vi "Processing Loop.vi"   [LabVIEW 2014, in "navX Library v2.lvlib"]
uses:
  navX Library v2.lvlib
  TypeDefs/navX Device TypeDef.ctl
  TypeDefs/navX Protocol TypeDef.ctl
  TypeDefs/navX Notify Packet TypeDef.ctl
  TypeDefs/navX Action TypeDef.ctl
  <vilib>/Platform/TimedLoop/XDataNode/timing_clust.ctl
  <vilib>/Platform/TimedLoop/XDataNode/nitl_modes.ctl
  <vilib>/Platform/TimedLoop/XDataNode/wakeup.ctl
  <vilib>/platform/TimedLoop/XDataNode/XDataNode.xnode
  <vilib>/Platform/TimedLoop/XDataNode/XDNodeRunTimeDep.lvlib
types:
  T1 = typedef "navX Library v2.lvlib/navX Device TypeDef.ctl" = cluster{"Interface":cluster{"Protocol":T2, "Update Rate (4Hz-60Hz)":u8, "navX Open TypeDef":variant}, "Notifiy Packet":refnum<notifier>, "Loop VI Refnum":refnum<vi>}
  T2 = typedef "navX Library v2.lvlib/navX Protocol TypeDef.ctl" = enum16{"SERIAL", "I2C", "SPI"}
  T3 = typedef "navX Library v2.lvlib/navX Interface TypeDef.ctl" = cluster{"SerialPortRef":T4, "I2CDevRef":T5, "SPIDevRef":T8}
  T4 = typedef "WPI_SerialPortRef.ctl" = cluster{"DevStatus":errorcluster, "Serial Port Name":refnum<visa-resource-name>}
  T5 = typedef "WPI_I2CDevRef.ctl" = cluster{"DevStatus":errorcluster, "Controller":T6, "Device Address":u8, "Handle":i32, "I2C Bus":T7}
  T6 = typedef "FPGA_TypedefDigitalModule.ctl" = enum16{"Controller 1"}
  T7 = typedef "i2c_bus.ctl" = enum16{"I2C On-Board", "I2C MXP", "Invalid"}
  T8 = typedef "WPI_SPIDevRef.ctl" = cluster{"DevStatus":errorcluster, "Handle":i32, "Controller":T6, "SPI Bus":T9}
  T9 = typedef "spi_bus.ctl" = enum16{"SPI On-Board, CS0", "SPI On-Board, CS1", "SPI On-Board, CS2", "SPI On-Board, CS3", "SPI MXP", "Invalid"}
  T10 = typedef "XDNodeRunTimeDep.lvlib/timing_clust.ctl" = cluster{"Expected End [f-1]":u64, "Actual End [f-1]":u64, "Finished Late? [f-1]":bool, "Expected End [i-1]":u64, "Actual End [i-1]":u64, "Finished Late? [i-1]":bool, "Expected Start [i]":u64, "Actual Start [i]":u64, "Expected Start [f]":u64, "Actual Start [f]":u64, "Source Name":string, "Structure Name":string, "Period":i64, "Deadline":i64, "Offset":i64, "Start":i64, "Priority":i32, "Timeout":i32, "Mode":T11, "Wakeup Reason":T12, "Error":errorcluster, "Source Type":string, "Secondary Source Type":string, "Global End Time":u64, "Global Start Time":u64, "Frame Duration":u64, "Iteration Duration":u64, "Assigned CPU":i32, "I/O Scan Engine Mode":u32}
  T11 = typedef "XDNodeRunTimeDep.lvlib/nitl_modes.ctl" = enum32{"No Change", "Process missed periods, maintain original phase", "Discard missed periods, maintain original phase", "Process missed periods, ignore original phase", "Discard missed periods, ignore original phase"}
  T12 = typedef "XDNodeRunTimeDep.lvlib/wakeup.ctl" = enum32{"Normal", "Aborted", "Asynchronous wakeup", "Timing source error", "Timed loop error", "Timeout"}
  T13 = typedef "navX Library v2.lvlib/navX Notify Packet TypeDef.ctl" = cluster{"navX Action":T14, "Data":variant}
  T14 = typedef "navX Library v2.lvlib/navX Action TypeDef.ctl" = enum16{"None", "Halt", "Reboot Detected", "Zero-Yaw"}
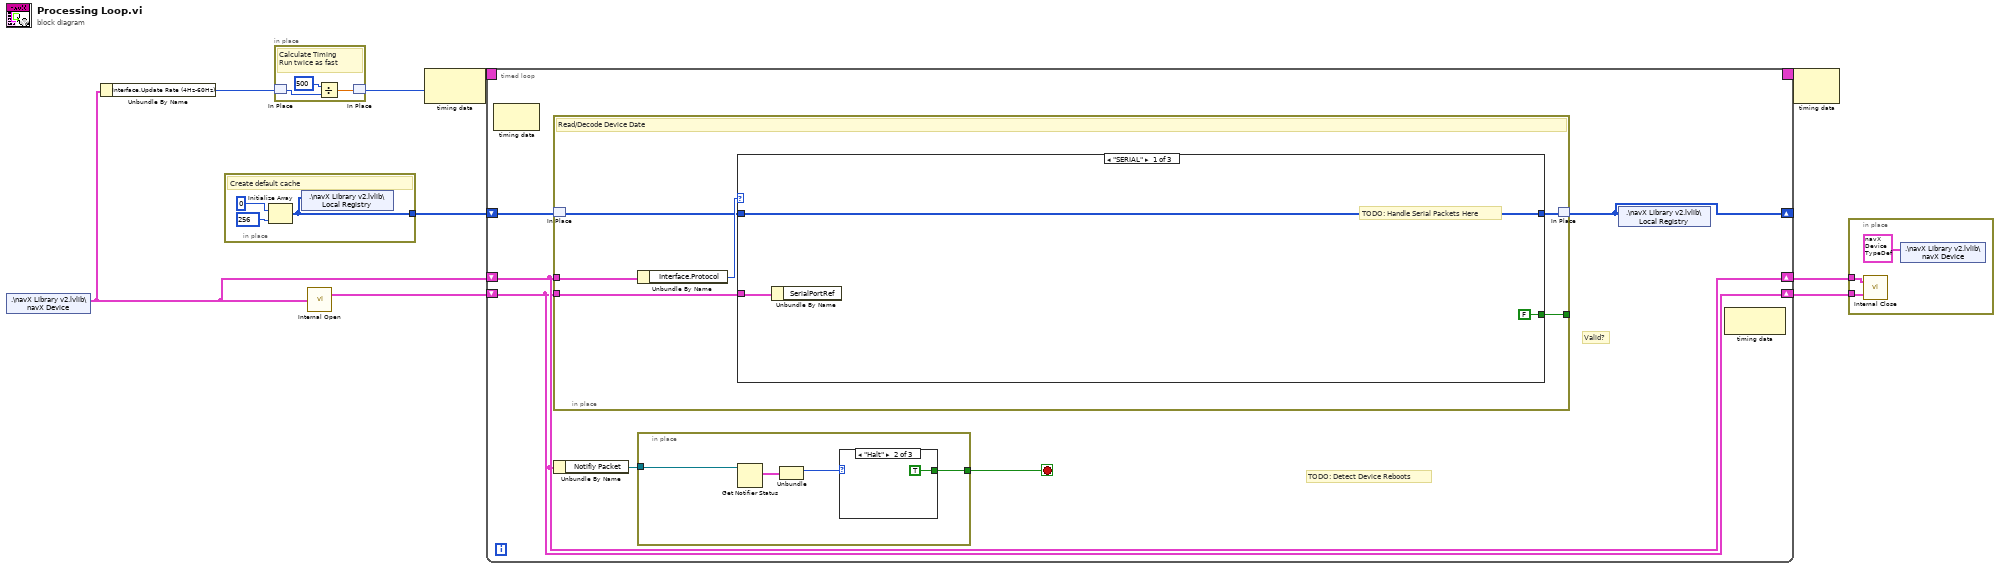
[diagram p0: block diagram]
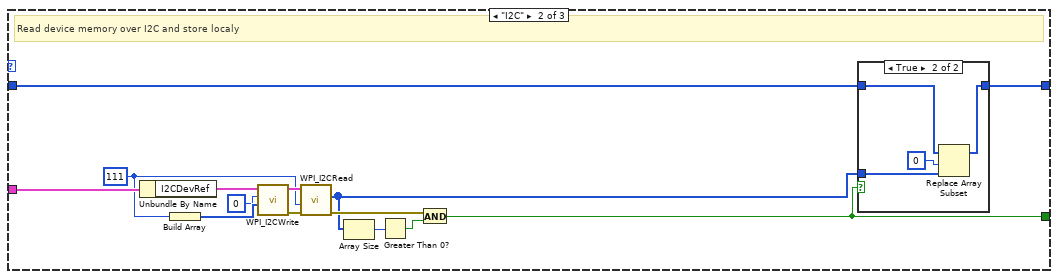
[diagram p2: hidden frame]
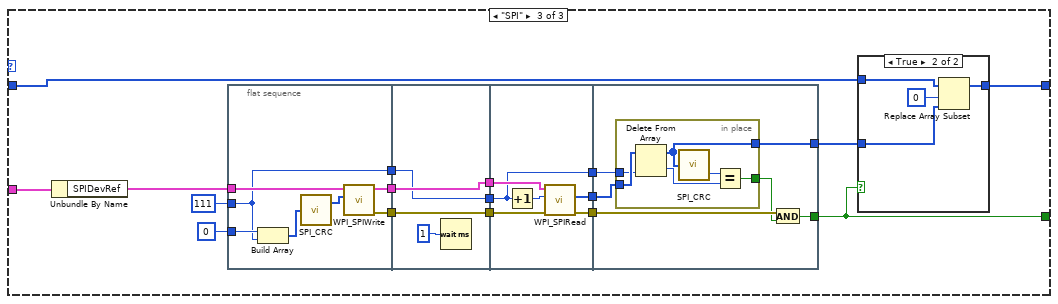
[diagram p4: hidden frame]
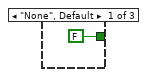
[diagram p6: hidden frame]
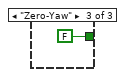
[diagram p7: hidden frame]
diagram:
  n1 = shared-variable ".\\navX Library v2.lvlib\\navX Device"() -> (w2:T1)  [unwired: 1 in, 1 out]
  n2 = Unbundle By Name(w2) -> ("Interface.Update Rate (4Hz-60Hz)"=w6:u8)
  n3 = in-place {
    in-place-border: [w10] -> w5
    # "Create default cache"
    n4 = Initialize Array(u8 0 ("Received Data"), 256 ("hex")) -> (w10:u8[])
    n5 = shared-variable ".\\navX Library v2.lvlib\\Local Registry"(w10) -> ()  [unwired: 1 in, 1 out]
  }
  n6 = in-place {
    # "Calculate Timing\nRun twice as fast"
    n7 = in-place-match #1(w6) -> (w14:u8)
    n8 = Divide(x=500, y=w14) -> (x/y=w13:dbl)
    n9 = in-place-match #1(w13) -> (w7:u8)
  }
  n10 = call "Internal Open.vi"("navX Device"=w2) -> ("Interface TypeDefs"=w1:T3)  [unwired: 1 out]
  n11 = node-c288(w7) -> (w9:T10)
  n12 = timed-loop {
    timing: w9 -> [_]
    timing-out: [_] -> w8
    shift-right: [w17] -> _
    shift-left: w5 -> [w18]
    shift-right: [w19] -> w4
    shift-left: w2 -> [w19]
    shift-right: [w16] -> w3
    shift-left: w1 -> [w16]
    stop <- w21 stop-if-true
    # "TODO: Detect Device Reboots"
    # "Valid?"
    n13 = node-c288() -> ()  [unwired: 1 in, 1 out]
    n14 = in-place {
      in-place-border: w19 -> [w27]
      in-place-border: w16 -> [w25]
      in-place-border: [w23] -> _
      # "Read/Decode Device Date"
      n15 = in-place-match #2(w18) -> (w24:u8[])
      n16 = Unbundle By Name(w27) -> ("Interface.Protocol"=w26:T2)
      n17 = case shown="\"SERIAL\"" w26 {
        tunnel: [w30 w32 w56] -> w22
        tunnel: w24 -> [w30 w34 w66]
        tunnel: w25 -> [w29 w44 w65]
        tunnel: [FALSE w31 w53] -> w23
        frame "SERIAL" {
          # "TODO: Handle Serial Packets Here"
          n18 = Unbundle By Name(w29) -> ()  [unwired: 1 out]
        }
        frame "I2C" {
          w39 = u8 111 ("hex")
          # "Read device memory over I2C and store localy"
          n19 = Unbundle By Name(w44) -> ("I2CDevRef"=w43:T5)
          n20 = Build Array(w39) -> (w42:u8[])
          n21 = call <vilib>:"WPI_I2CWrite.vi"("I2CDataToSend"=w42, "I2CRegister"=u8 0 ("hex"), "I2CDevRef"=w43) -> ("error out"=w41:errorcluster, "I2CDevRef"=w40:T5)  [unwired: 7 in]
          n22 = call <vilib>:"WPI_I2CRead.vi"("error in (no error)"=w41, "I2CBytesToRead"=w39, "I2CDevRef"=w40) -> ("error out"=w35:errorcluster, "Data Out"=w33:u8[])  [unwired: 6 in, 1 out]
          n23 = Array Size(array=w33) -> (size(s)=w37:i32)
          n24 = Greater Than 0?(x=w37) -> (x > 0?=w36:bool)
          n25 = And(x=w35, y=w36) -> (x .and. y?=w31:bool)
          n26 = case shown="True" w31 {
            tunnel: w34 -> [w45 w49]
            tunnel: [w45 w48] -> w32
            tunnel: w33 -> [_ w47]
            frame False {
            }
            frame True {
              n27 = Replace Array Subset(array=w49, new element=w47, index=u8 0 ("hex")) -> (w48:u8[])
            }
          }
        }
        frame "SPI" {
          n28 = Unbundle By Name(w65) -> ("SPIDevRef"=w63:T8)
          n29 = flat-sequence {
            tunnel: u8 0 ("hex") -> [w78]
            tunnel: u8 111 ("hex") -> [w73]
            tunnel: w63 -> [w75]
            tunnel: [w74] -> w62
            tunnel: [w73] -> w59
            tunnel: [w72] -> w52
            tunnel: w62 -> [w81]
            tunnel: [w81] -> w61
            tunnel: [w80] -> w60
            tunnel: w59 -> [w80]
            tunnel: w52 -> [w79]
            tunnel: [w79] -> w51
            tunnel: w61 -> [w88]
            tunnel: w60 -> [w85]
            tunnel: [w86] -> w58
            tunnel: [w85] -> w57
            tunnel: w51 -> [w84]
            tunnel: [w83] -> w50
            tunnel: w58 -> [w94]
            tunnel: w57 -> [w93]
            tunnel: [w89] -> w53
            tunnel: [w92] -> w55
            tunnel: w50 -> [w91]
            frame #0 {
              n30 = Build Array(w78, w73) -> (w77:u8[])
              n31 = call "SPI_CRC.vi"("Message"=w77) -> ("Message with CRC"=w76:u8[])  [unwired: 1 out]
              n32 = call <vilib>:"WPI_SPIWrite.vi"("Data To Send"=w76, "SPIDevRef"=w75) -> ("error out"=w72:errorcluster, "SPIDevRef"=w74:T8)  [unwired: 7 in, 1 out]
            }
            frame #1 {
              n33 = Wait (ms)(milliseconds to wait=u32 1) -> ()  [unwired: 1 out]
            }
            frame #2 {
              n34 = Increment(x=w85) -> (x+1=w87:u8)
              n35 = call <vilib>:"WPI_SPIRead.vi"("error in (no error)"=w84, "Num to Read"=w87, "SPIDevRef"=w88) -> ("error out"=w83:errorcluster, "Received Data"=w86:u8[])  [unwired: 6 in, 1 out]
            }
            frame #3 {
              n36 = in-place {
                in-place-border: w94 -> [w100]
                in-place-border: w93 -> [w99]
                in-place-border: [w96] -> w90
                in-place-border: [w95] -> w92
                n37 = Delete From Array(array=w100, index=w99) -> (deleted portion=w98:u8, array with subset deleted=w95:u8[])  [unwired: 1 in]
                n38 = call "SPI_CRC.vi"("Message"=w95) -> ("CRC"=w97:u8)  [unwired: 1 out]
                n39 = Equal?(x=w97, y=w98) -> (x = y?=w96:bool)
              }
              n40 = And(x=w91, y=w90) -> (x .and. y?=w89:bool)
            }
          }
          n41 = case shown="True" w53 {
            tunnel: w66 -> [w67 w71]
            tunnel: [w67 w70] -> w56
            tunnel: w55 -> [_ w69]
            frame False {
            }
            frame True {
              n42 = Replace Array Subset(array=w71, new element=w69, index=u8 0 ("hex")) -> (w70:u8[])
            }
          }
        }
      }
      n43 = in-place-match #2(w22) -> (w17:u8[])
    }
    n44 = Unbundle By Name(w19) -> ("Notifiy Packet"=w20:refnum<notifier>)
    n45 = in-place {
      in-place-border: [w102] -> w21
      in-place-border: w20 -> [w101]
      n46 = Get Notifier Status(notifier=w101) -> (current notification=w104:T13)  [unwired: 1 in, 4 out]
      n47 = Unbundle(w104) -> ("navX Action"=w103:T14)  [unwired: 1 out]
      n48 = case shown="\"Halt\"" w103 {
        tunnel: [FALSE TRUE FALSE] -> w102
        frame "None", Default {
        }
        frame "Halt" {
        }
        frame "Zero-Yaw" {
        }
      }
    }
    n49 = shared-variable ".\\navX Library v2.lvlib\\Local Registry"(w17) -> ()  [unwired: 1 in, 1 out]
    n50 = node-c288() -> ()  [unwired: 1 in, 1 out]
  }
  n51 = node-c288(w8) -> ()  [unwired: 1 out]
  n52 = in-place {
    in-place-border: w4 -> [w112]
    in-place-border: w3 -> [w111]
    n53 = call "Internal Close.vi"("Interface TypeDefs"=w111, "navX Device"=w112) -> ()  [unwired: 1 out]
    n54 = shared-variable ".\\navX Library v2.lvlib\\navX Device"(T1 {"Interface"={"Protocol"=enum."SERIAL", "Update Rate (4Hz-60Hz)"=4, "navX Open TypeDef"=variant}, "Notifiy Packet"=refnum, "Loop VI Refnum"=refnum} ("navX Device")) -> ()  [unwired: 1 in, 1 out]
  }
